vi "Set Control List State.vi"(8 "error in (no error)":errorcluster, 10 "Control List":string[](array[string])=["Ramp to Zero", "Crowbar", "Read FPGA Config", "Clear Quench"], 11 "Enable Disable":T1(ring)) -> (0 "error out":errorcluster)   [LabVIEW 2019]
doc: "Author: Scott Hannahs <sth@magnet.fsu.edu>\nCopyright 2018 Florida State University, All rights reserved."
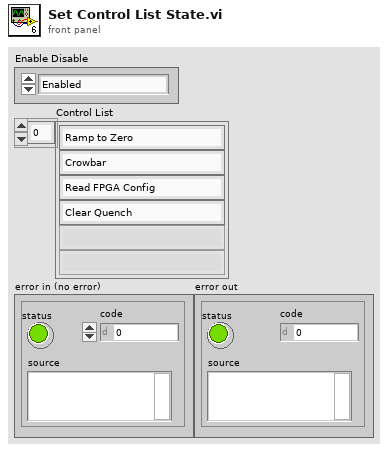
[diagram p1: front panel]
types:
  T1 = enum8{"Enabled", "Disabled", "Disabled and Grayed Out"}
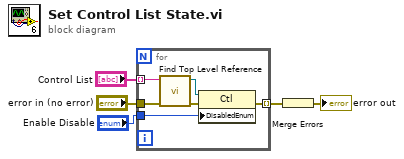
[diagram p0: block diagram]
diagram:
  n1 = for {
    tunnel: "Enable Disable" -> [w10]
    tunnel: "Control List" -> [w8] mode=indexing
    tunnel: [w7] -> w3 mode=indexing
    tunnel: "error in (no error)" -> [w6]
    n2 = call "Find Top Level Reference.vi"("error in (no error)"=w6, "String"=w8) -> ("error out"=w9:errorcluster, "Ctl Refnum"=w11:refnum<vi>)  [unwired: 8 in]
    n3 = property on="Property Node" class="Ctl"(reference=w11, error in=w9, "DisabledEnum"=w10) -> (error out=w7:errorcluster)  [unwired: 1 out]
  }
  n4 = Merge Errors(w3) -> (→"error out":errorcluster)
